vi "C867_Macro.vi"(8 "error in":errorcluster caption="entrée d'erreur") -> (0 "error out":errorcluster caption="sortie d'erreur")   [LabVIEW 2026]
uses:
  Controls/TypeDef_FGV.ctl
panel:
  out "szCommand out":string
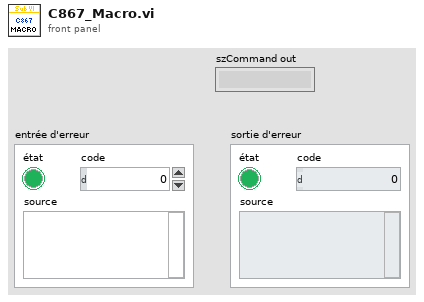
[diagram p1: front panel]
types:
  T1 = typedef "TypeDef_FGV.ctl" = enum16{"Initialize", "Write", "Read"}
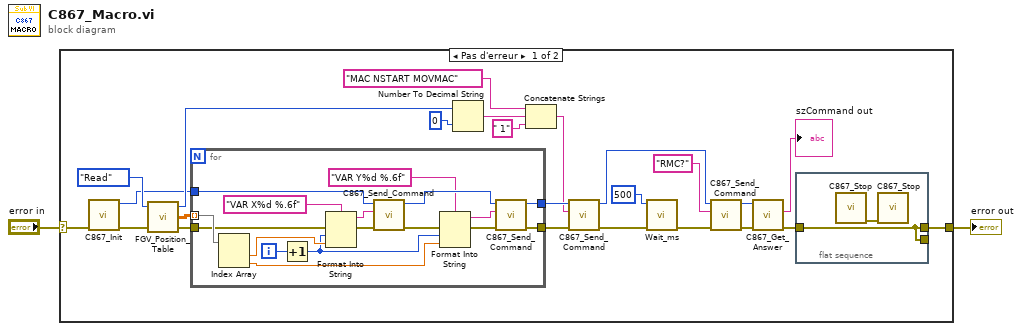
[diagram p0: block diagram]
diagram:
  n1 = case shown="Pas d'erreur" "error in" {
    selector: "error in" -> [w17 w46]
    tunnel: [w10 w46] -> w1
    frame No Error {
      n2 = call "C867_Init.vi"("error in"=w17) -> ("error out"=w16:errorcluster, "ID"=w15:i32)  [unwired: 9 in]
      n3 = call "FGV_Position_Table.vi"("error in"=w16, "Action"=TypeDef_FGV."Read") -> ("error out"=w26:errorcluster, "Position table"=w25:dbl[][], "N pos"=w21:i32)  [unwired: 1 in]
      n4 = for {
        tunnel: w25 -> [w45] mode=indexing
        tunnel: w26 -> [w44]
        tunnel: w15 -> [w37]
        tunnel: [w30] -> w14
        tunnel: [w29] -> w12
        i -> [w34]
        n5 = Index Array(array=w45) -> (element #1=w35:dbl, element #2=w32:dbl)  [unwired: 2 in]
        n6 = Increment(x=w34) -> (x+1=w31:i32)
        n7 = Format Into String(format string="VAR X%d %.6f" ("chaîne initiale"), error in=w44, w31, w35) -> (resulting string=w42:string, error out=w41:errorcluster)  [unwired: 1 in]
        n8 = call "C867_Send_Command.vi"("entrée d'erreur (pas d'erreur)"=w41, "szCommand"=w42, "ID en entrée"=w37) -> ("sortie d'erreur"=w38:errorcluster, "ID en sortie"=w36:i32)  [unwired: 5 in, 2 out]
        n9 = Format Into String(format string="VAR Y%d %.6f" ("chaîne initiale"), error in=w38, w31, w32) -> (resulting string=w39:string, error out=w40:errorcluster)  [unwired: 1 in]
        n10 = call "C867_Send_Command.vi"("entrée d'erreur (pas d'erreur)"=w40, "szCommand"=w39, "ID en entrée"=w36) -> ("sortie d'erreur"=w30:errorcluster, "ID en sortie"=w29:i32)  [unwired: 5 in, 2 out]
      }
      n11 = Number To Decimal String(number=w21, width (-)=i16 0 ("largeur (-)")) -> (decimal integer string=w20:string)
      n12 = Concatenate Strings("MAC NSTART MOVMAC", w20, " 1" ("chaîne")) -> (w11:string)
      n13 = call "C867_Send_Command.vi"("entrée d'erreur (pas d'erreur)"=w14, "szCommand"=w11, "ID en entrée"=w12) -> ("sortie d'erreur"=w13:errorcluster, "ID en sortie"=w8:i32)  [unwired: 5 in, 2 out]
      n14 = call "Wait_ms.vi"("error in (no error)"=w13, "milliseconds to wait"=u32 500) -> ("error out"=w9:errorcluster)  [unwired: 9 in]
      n15 = call "C867_Send_Command.vi"("entrée d'erreur (pas d'erreur)"=w9, "szCommand"="RMC?", "ID en entrée"=w8) -> ("sortie d'erreur"=w5:errorcluster, "ID en sortie"=w6:i32)  [unwired: 5 in, 2 out]
      n16 = call "C867_Get_Answer.vi"("entrée d'erreur (pas d'erreur)"=w5, "ID en entrée"=w6) -> ("sortie d'erreur"=w4:errorcluster, "szAnswer"=→"szCommand out":string)  [unwired: 6 in, 2 out]
      n17 = flat-sequence {
        tunnel: [w27] -> w10
        tunnel: [w27] -> _
        tunnel: w4 -> [w27]
        frame #0 {
          n18 = call "C867_Stop.vi"() -> ("error out"=w28:errorcluster)  [unwired: 11 in]
          n19 = call "C867_Stop.vi"("error in"=w28) -> ()  [unwired: 10 in, 1 out]
        }
      }
    }
    frame Error {
    }
  }
  "error out" <- w1
